vi "ADC.vi"(0 "Bits":i32, 5 "Channels":i32, 7 "Sampling rate":i32, 11 "Error in":errorcluster) -> (4 "Digital 1D":u8[](array[numeric]), 6 "Analog Data":dbl[](array[numeric]), 15 "Error out":errorcluster)   [LabVIEW 2020, in "ADC_MultiChannel.lvlib"]
doc: "This VI is used in generating Analog data and converting the same to digital and sends the data as 1D U8 array."
uses:
  ADC_MultiChannel.lvlib
  <vilib>/numeric/Random Number (Range) DBL.vi
panel:
  in  "Vref":dbl=5.0
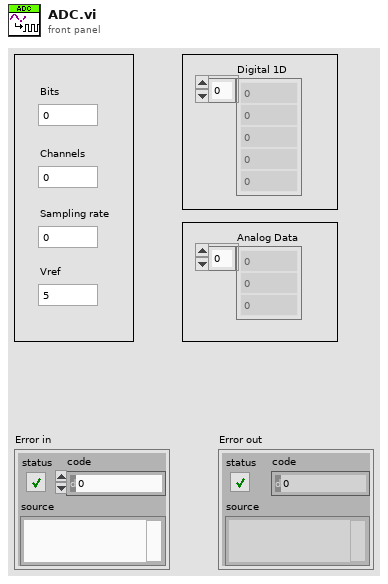
[diagram p1: front panel]
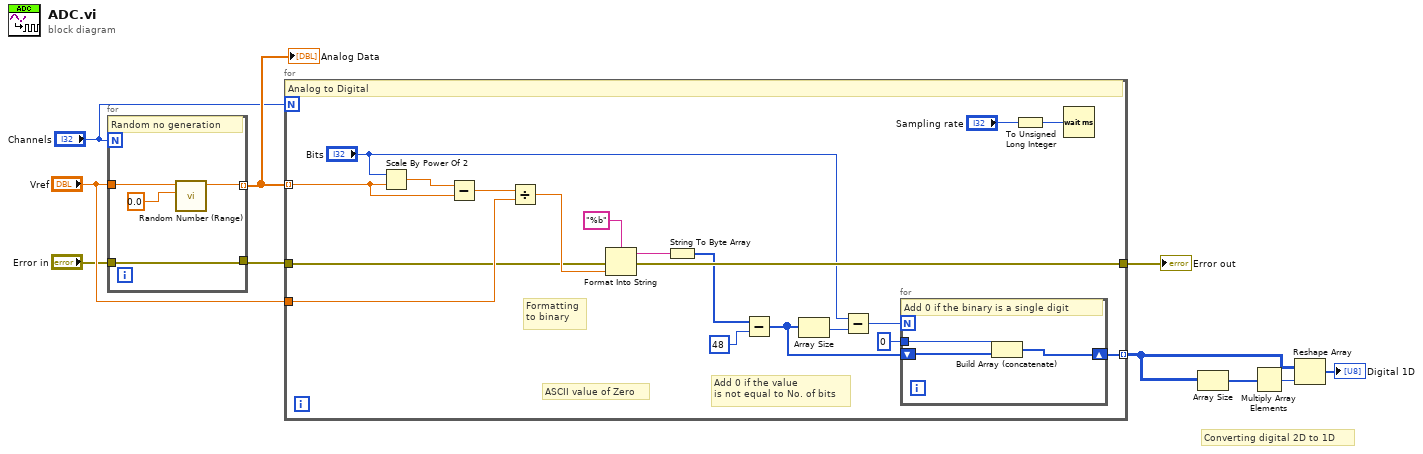
[diagram p0: block diagram]
diagram:
  # "Converting digital 2D to 1D"
  n1 = for {
    N: "Channels" -> [_]
    tunnel: "Vref" -> [w14]
    tunnel: [w12] -> w10 mode=indexing
    tunnel: "Error in" -> [w11]
    tunnel: [w11] -> w6
    # "Random no generation"
    n2 = call-poly <vilib>:"Random Number (Range).vi"("lower bound (0)"=0.0, "upper bound (100)"=w14) -> ("number"=w12:dbl)  [unwired: 9 in]
  }
  "Analog Data" <- w10
  n3 = for {
    N: "Channels" -> [_]
    tunnel: w10 -> [w32] mode=indexing
    tunnel: "Vref" -> [w30]
    tunnel: [w27] -> w8
    tunnel: w6 -> [w26]
    tunnel: [w17] -> w3 mode=indexing
    # "Add 0 if the value\nis not equal to No. of bits"
    # "ASCII value of Zero"
    # "Formatting\nto binary"
    # "Analog to Digital"
    n4 = Scale By Power Of 2(n="Bits", x=w32) -> (x*2^n=w33:dbl)
    n5 = Subtract(x=w33, y=w32) -> (x-y=w31:dbl)
    n6 = Divide(x=w31, y=w30) -> (x/y=w28:dbl)
    n7 = Format Into String(format string="%b", error in=w26, w28) -> (resulting string=w25:string, error out=w27:errorcluster)  [unwired: 1 in]
    n8 = String To Byte Array(string=w25) -> (unsigned byte array=w24:u8[])
    n9 = Subtract(x=w24, y=u8 48) -> (x-y=w19:u8[])
    n10 = Array Size(array=w19) -> (size(s)=w22:i32)
    n11 = Subtract(x="Bits", y=w22) -> (x-y=w20:i32)
    n12 = for {
      N: w20 -> [_]
      shift-right: [w34] -> w17
      shift-left: w19 -> [w36]
      tunnel: u8 0 -> [w35]
      # "Add 0 if the binary is a single digit"
      n13 = Build Array (concatenate)(w35, w36) -> (w34:u8[])
    }
    n14 = To Unsigned Long Integer(number="Sampling rate") -> (unsigned 32bit integer=w15:u32)
    n15 = Wait (ms)(milliseconds to wait=w15) -> ()  [unwired: 1 out]
  }
  "Error out" <- w8
  n16 = Array Size(array=w3) -> (size(s)=w5:i32[])
  n17 = Multiply Array Elements(1:w5) -> (0:w4:i32)
  n18 = Reshape Array(w3, w4) -> (→"Digital 1D":u8[])
